vi "Vision Processing.vi"(4 "error in (no error)":errorcluster, 7 "Image Size":T5=enum."320x240") -> ()   [LabVIEW 2015]
uses:
  <vilib>/Rock Robotics/WPI/Camera/WPI_CameraImageSize.ctl
  <vilib>/Rock Robotics/WPI/Camera/WPI_CameraWhite Balance Values.ctl
  <vilib>/Rock Robotics/WPI/Camera/WPI_CameraExposure Values.ctl
  <vilib>/Rock Robotics/WPI/Camera/WPI_CameraFrameRate.ctl
  Vision Support Code/Camera Types.ctl
  Robot Global Data.vi
  <vilib>/vision/NI_Vision_Development_Module.lvlib
panel:
  out "Normalized Rect":T1
  out "Center":cluster{dbl, dbl}
  out "element":T2
  out "Highest Avg Score":dbl
  in  "Min Score Threshold":i32=75
  out "Detected Targets":T3(array[cluster]) {"Normalized Rect"."Numeric 5" format="%#_2g"; "Normalized Rect"."Numeric 3" format="%#_2g"; "Normalized Rect"."Numeric 2" format="%#_2g"; "Normalized Rect"."Numeric" format="%#_2g"}
  out "Sorted Particle Scores":T4(array[cluster]) {"Moment Factor" format="%#_3g"; "Aspect Ratio" format="%#_3g"; "Area to CH" format="%#_3g"; "X" format="%#_3g"; "Y" format="%#_3g"}
  in  "Display Original":bool=TRUE
  in  "Display Mask":bool=TRUE
  out "fps":dbl
  in  "Emphasize Limit Tests":bool=TRUE
  in  "Aspect Fudge Factor":dbl=1.0
  in  "Score Threshold":dbl=75.0
  out "ms to process":u32
  out "Qualified Particles":i32
  in  "LED Color":T6={"Hue"={111.0, 149.0}, "Sat"={35.0, 255.0}, "Val"={93.0, 255.0}} {"Hue" scale=0.0..255.0 scale format="%#_3g"}
  out "Masked":T7(plugin-control)
  out "Original Image":T7(plugin-control)
  # "NOTE:\nFor best results, lower the camera\nexposure."
  # "This is only the initial camera size.\nOther camera setup is done\non the diagram. Notice it is set\nonce before the loop but can be\nupdated within the loop if needed."
  # "Instructions:\nUse LED Color to threshold and build particles. Adjust calibration if needed.\nDisplays are very useful for debugging, but will slow down execution, so you\nmay want to disable once working.\nAnnotations show the rectangle and the scores from top to bottom.\nChange camera setting on diagram."
  # "Density Profile"
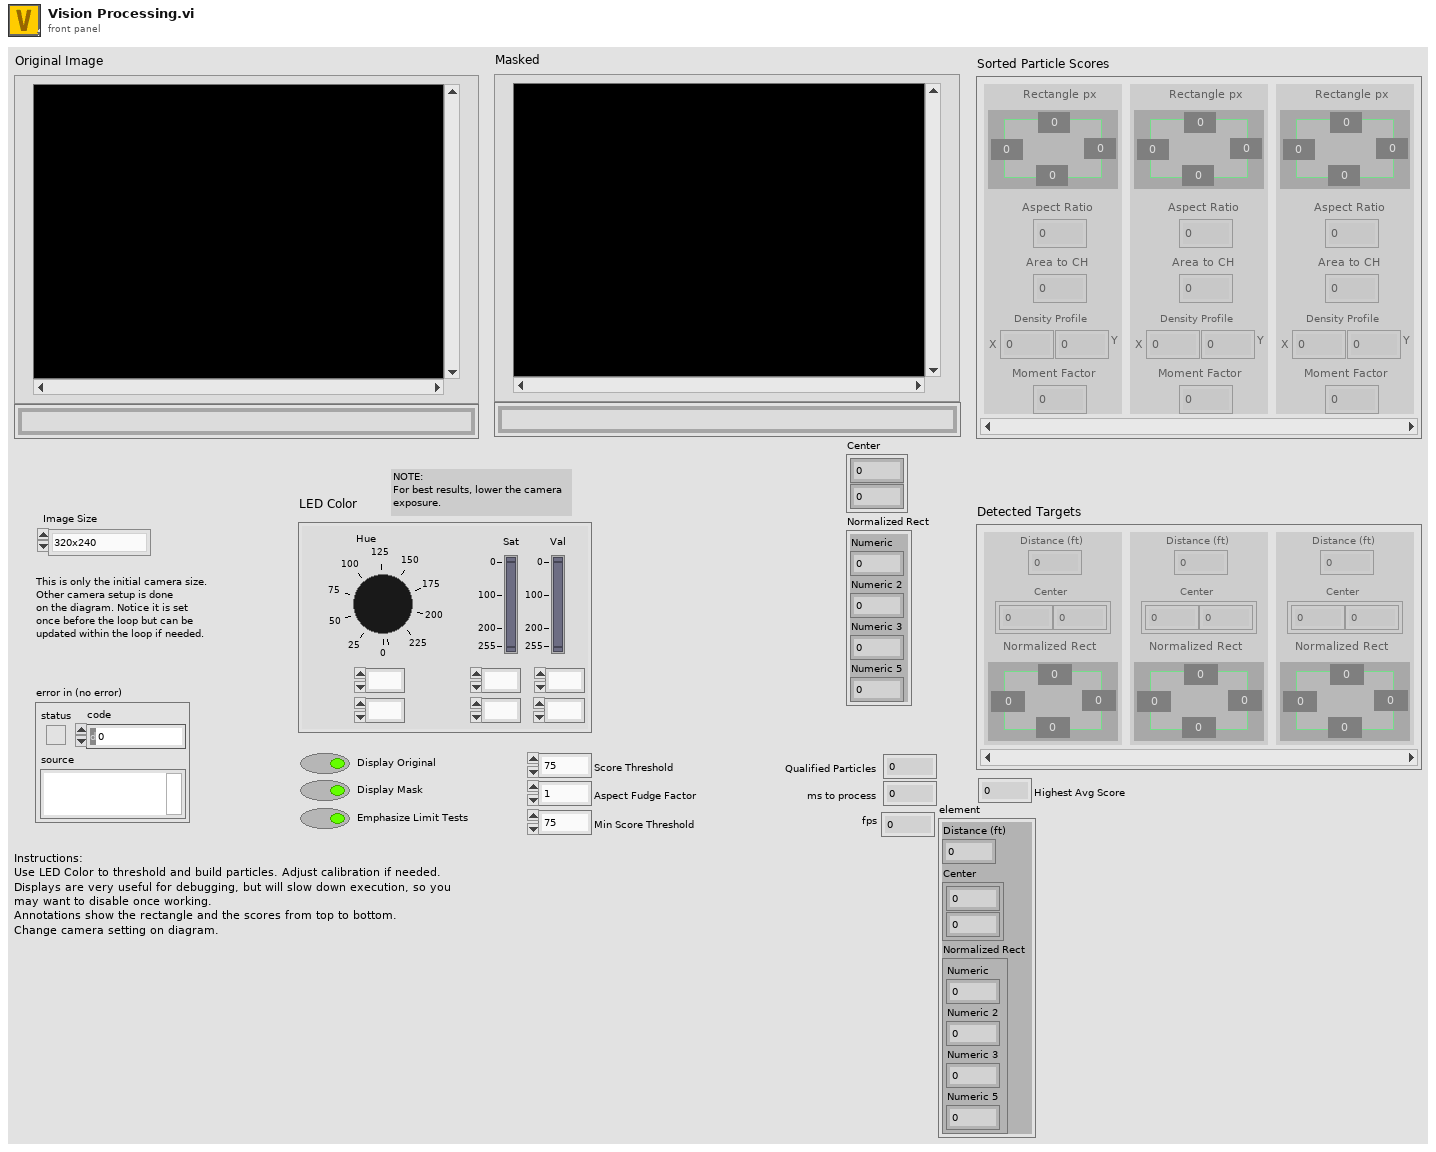
[diagram p1: front panel]
types:
  T1 = cluster{"Numeric":dbl, "Numeric 2":dbl, "Numeric 3":dbl, "Numeric 5":dbl}
  T2 = cluster{"Distance (ft)":dbl, "Center":cluster{dbl, dbl}, "Normalized Rect":cluster{"Numeric":dbl, "Numeric 2":dbl, "Numeric 3":dbl, "Numeric 5":dbl}}
  T3 = cluster{"Distance (ft)":dbl, "Center":cluster{dbl, dbl}, "Normalized Rect":cluster{"Numeric":dbl, "Numeric 2":dbl, "Numeric 3":dbl, "Numeric 5":dbl}}[]
  T4 = cluster{"Rectangle px":cluster{"Numeric":dbl, "Numeric 2":dbl, "Numeric 3":dbl, "Numeric 5":dbl}, "Aspect Ratio":dbl, "Area to CH":dbl, "X":dbl, "Y":dbl, "Moment Factor":dbl}[]
  T5 = typedef "WPI_CameraImageSize.ctl" = enum16{"640x480", "320x240", "160x120", "Custom"}
  T6 = cluster{"Hue":cluster{dbl, dbl}, "Sat":cluster{dbl, dbl}, "Val":cluster{dbl, dbl}}
  T7 = typedef "IMAQ Image.ctl" = refnum<image>
  T8 = typedef "WPI_CameraFrameRate.ctl" = u32
  T9 = typedef "WPI_CameraExposure Values.ctl" = enum16{"Auto", "Flicker-free 50 Hz", "Flicker-free 60 Hz", "Hold current", "Custom"}
  T10 = typedef "WPI_CameraWhite Balance Values.ctl" = enum16{"Auto", "Fixed indoor", "Fixed outdoor 1", "Fixed outdoor 2", "Fixed fluorescent 1", "Fixed fluorescent 2", "Hold current", "Custom"}
  T11 = typedef "Particle Parameters" = i32
  T12 = typedef "Image Type" = u32
  T13 = typedef "WPI_CameraDevRef.ctl" = cluster{"Camera Address":string, "CameraStatus":errorcluster}
  T14 = typedef "Camera Types.ctl" = enum16{"206", "1011", "1013", "MS HD3000 square", "MS HD3000 640x480"}
  T15 = cluster{"Bounding box":cluster{"left":dbl, "top":dbl, "right":dbl, "bottom":dbl}, "Aspect Ratio":dbl, "Area to CH":dbl, "X Mask":dbl, "Y Mask":dbl, "Moment":dbl}[]
  T16 = cluster{"Rectangle":cluster{"Numeric":dbl, "Numeric 2":dbl, "Numeric 3":dbl, "Numeric 5":dbl}, "L":dbl, "Area to CH":dbl, "X":dbl, "Y":dbl, "Moment Factor":dbl}[]
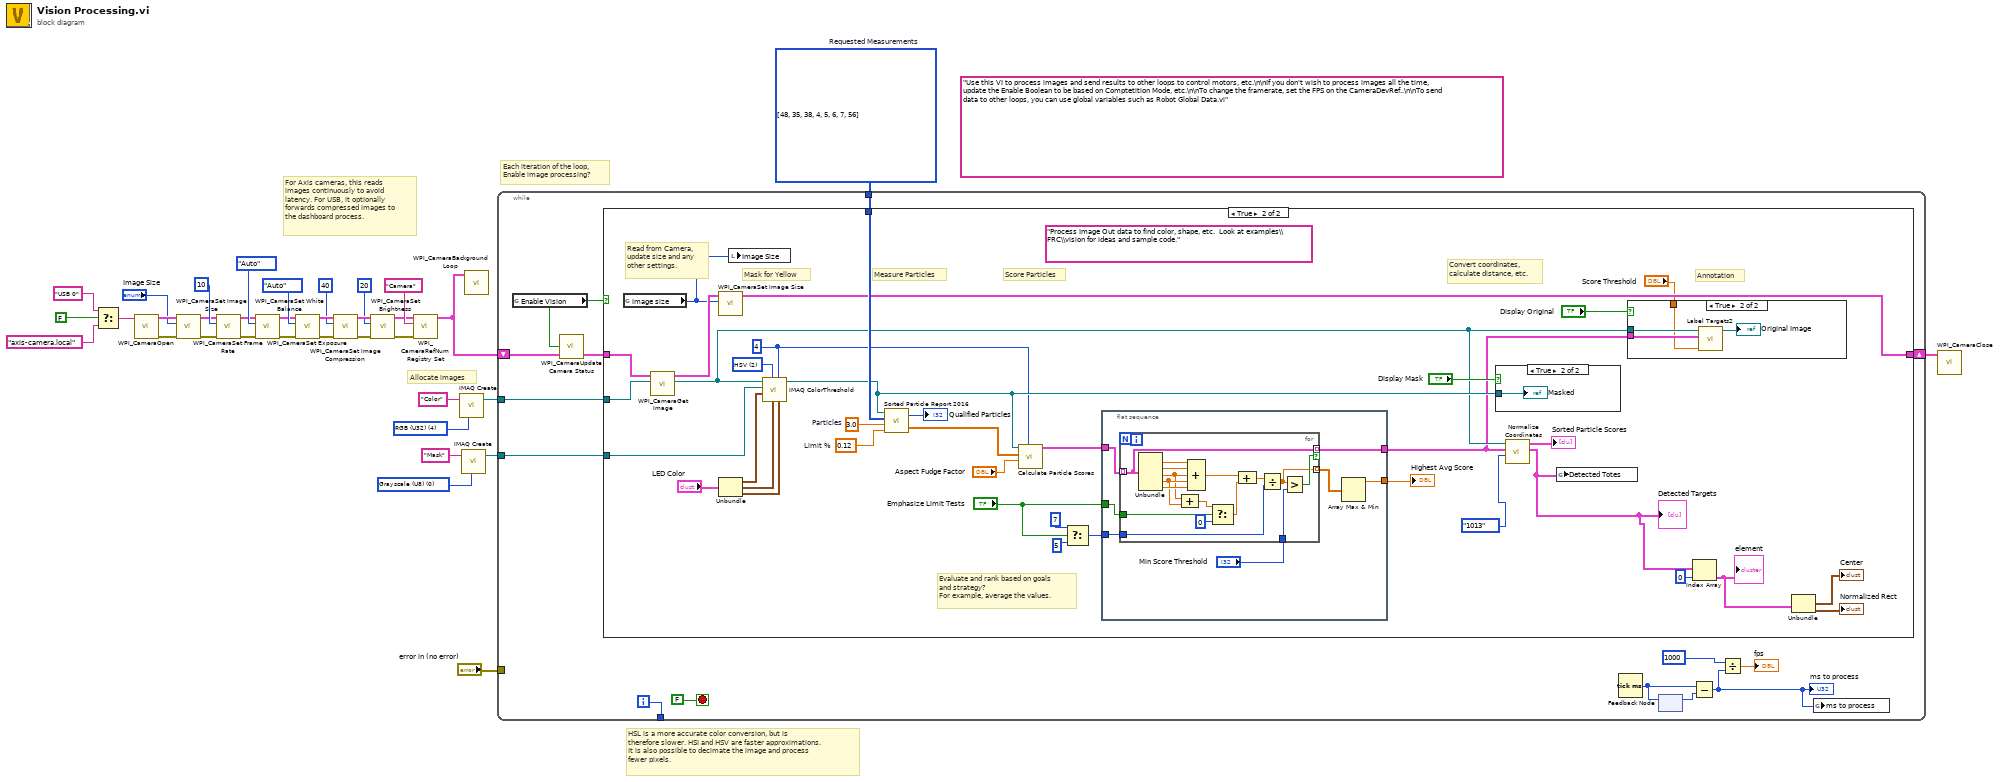
[diagram p0: block diagram]
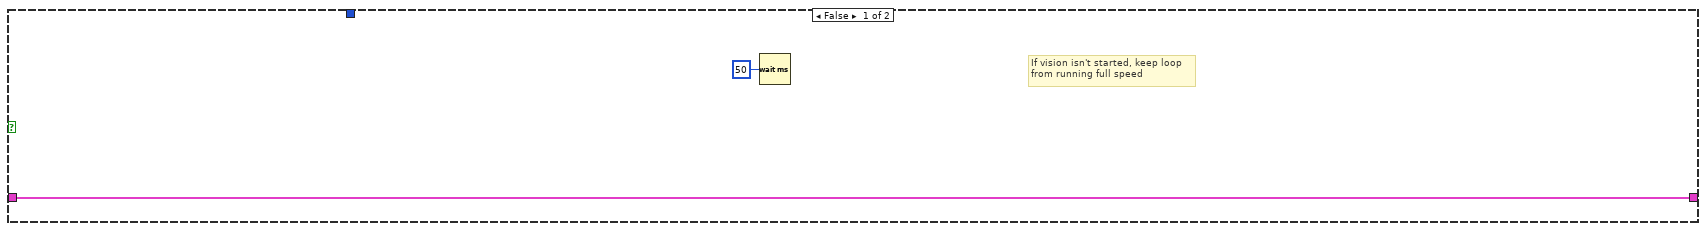
[diagram p2: hidden frame]
diagram:
  (unwired) "Use this VI to process images and send results to other loops to control motors, etc.\n\nIf you don't wish to process images all the time, update the Enable Boolean to be based on Comptetition Mode, etc.\n\nTo change the framerate, set the FPS on the CameraDevRef..\n\nTo send data to other loops, you can use global variables such as Robot Global Data.vi"
  w29 = T11[] [48, 35, 38, 4, 5, 6, 7, 56] items=["Center of Mass X", "Center of Mass Y", "First Pixel X", "First Pixel Y", "Bounding Rect Left", "Bounding Rect Top", "Bounding Rect Right", "Bounding Rect Bottom", "Max Feret Diameter Start X", "Max Feret Diameter Start Y", "Max Feret Diameter End X", "Max Feret Diameter End Y", "Max Horiz. Segment Length Left", "Max Horiz. Segment Length Right", "Max Horiz. Segment Length Row", "-", "Bounding Rect Width", "Bounding Rect Height", "Bounding Rect Diagonal", "Perimeter", "Convex Hull Perimeter", "Holes' Perimeter", "Max Feret Diameter", "Equivalent Ellipse Major Axis", "Equivalent Ellipse Minor Axis", "Equivalent Ellipse Minor Axis (Feret)", "Equivalent Rect Long Side", "Equivalent Rect Short Side", "Equivalent Rect Diagonal", "Equivalent Rect Short Side (Feret)", "Average Horiz. Segment Length", "Average Vert. Segment Length", "Hydraulic Radius", "Waddel Disk Diameter", "-", "Area", "Holes' Area", "Particle & Holes' Area", "Convex Hull Area", "Image Area", "-", "Number of Holes", "Number of Horiz. Segments", "Number of Vert. Segments", "-", "Orientation", "Max Feret Diameter Orientation", "-", "% Area/Image Area", "% Area/(Particle & Holes' Area)", "Ratio of Equivalent Ellipse Axes", "Ratio of Equivalent Rect Sides", "-", "Elongation Factor", "Compactness Factor", "Heywood Circularity Factor", "Type Factor", "-", "Sum X", "Sum Y", "Sum XX", "Sum XY", "Sum YY", "Sum XXX", "Sum XXY", "Sum XYY", "Sum YYY", "-", "Moment of Inertia XX", "Moment of Inertia XY", "Moment of Inertia YY", "Moment of Inertia XXX", "Moment of Inertia XXY", "Moment of Inertia XYY", "Moment of Inertia YYY", "Norm. Moment of Inertia XX", "Norm. Moment of Inertia XY", "Norm. Moment of Inertia YY", "Norm. Moment of Inertia XXX", "Norm. Moment of Inertia XXY", "Norm. Moment of Inertia XYY", "Norm. Moment of Inertia YYY", "Hu Moment 1", "Hu Moment 2", "Hu Moment 3", "Hu Moment 4", "Hu Moment 5", "Hu Moment 6", "Hu Moment 7"]  # Requested Measurements
  w32 = T12 0 items=["Grayscale (U8)", "Grayscale (I16)", "Grayscale (SGL)", "Complex (CSG)", "RGB (U32)", "HSL (U32)", "RGB (U64)", "Grayscale (U16)"] ("Image Type")
  w34 = T12 4 items=["Grayscale (U8)", "Grayscale (I16)", "Grayscale (SGL)", "Complex (CSG)", "RGB (U32)", "HSL (U32)", "RGB (U64)", "Grayscale (U16)"] ("Image Type")
  # "Each iteration of the loop,\nEnable image processing?"
  # "HSL is a more accurate color conversion, but is\ntherefore slower. HSI and HSV are faster approximations.\nIt is also possible to decimate the image and process\nfewer pixels."
  # "For Axis cameras, this reads\nimages continuously to avoid\nlatency. For USB, it optionally\nforwards compressed images to\nthe dashboard process."
  # "Allocate images"
  n1 = Select(t="USB 0" ("format string"), s=FALSE ("dot notation? (F)"), f="axis-camera.local" ("format string")) -> (s? t:f=w28:string)
  n2 = call <vilib>:"WPI_CameraOpen.vi"("Camera Address"=w28) -> ("error out"=w16:errorcluster, "CameraDevRef"=w15:T13)  [unwired: 1 in, 8 out]
  n3 = call <vilib>:"WPI_CameraSet Image Size.vi"("error in (no error)"=w16, "Image Size"="Image Size", "CameraDevRef"=w15) -> ("error out"=w17:errorcluster, "CameraDevRef Out"=w14:T13)  [unwired: 1 in, 6 out]
  n4 = call <vilib>:"WPI_CameraSet Frame Rate.vi"("error in (no error)"=w17, "Frame Rate (fps)"=T8 10, "CameraDevRef"=w14) -> ("error out"=w18:errorcluster, "CameraDevRef Out"=w12:T13)  [unwired: 7 out]
  n5 = call <vilib>:"WPI_CameraSet White Balance.vi"("error in (no error)"=w18, "White Balance"=WPI_CameraWhite_Balance_Values."Auto", "CameraDevRef"=w12) -> ("error out"=w19:errorcluster, "CameraDevRef Out"=w13:T13)  [unwired: 1 in, 6 out]
  n6 = call <vilib>:"WPI_CameraSet Exposure.vi"("error in (no error)"=w19, "Exposure"=WPI_CameraExposure_Values."Auto", "CameraDevRef"=w13) -> ("error out"=w20:errorcluster, "CameraDevRef Out"=w10:T13)  [unwired: 1 in, 6 out]
  n7 = call <vilib>:"WPI_CameraSet Image Compression.vi"("error in (no error)"=w20, "Compression"=40, "CameraDevRef"=w10) -> ("error out"=w21:errorcluster, "CameraDevRef Out"=w11:T13)  [unwired: 7 out]
  n8 = call <vilib>:"WPI_CameraSet Brightness.vi"("error in (no error)"=w21, "Brightness"=20, "CameraDevRef"=w11) -> ("error out"=w22:errorcluster, "CameraDevRef Out"=w1:T13)  [unwired: 7 out]
  n9 = call <vilib>:"WPI_CameraRefNum Registry Set.vi"("error in (no error)"=w22, "refnum name"="Camera", "CameraDevRef"=w1) -> ("CameraDevRef"=w6:T13)  [unwired: 1 in, 7 out]
  n10 = call "IMAQ Create"("Image Name"="Color", "Image Type"=w34) -> ("New Image"=w33:T7)  [unwired: 2 in, 2 out]
  n11 = call "IMAQ Create"("Image Name"="Mask", "Image Type"=w32) -> ("New Image"=w30:T7)  [unwired: 2 in, 2 out]
  n12 = call <vilib>:"WPI_CameraBackground Loop.vi"("CameraDevRef"=w6) -> ()  [unwired: 11 in]
  n13 = while {
    tunnel: w33 -> [w44]
    tunnel: w30 -> [w48]
    tunnel: w29 -> [w47]
    tunnel: "error in (no error)" -> [_]
    tunnel: [w43] -> _
    shift-right: [w39] -> w2
    shift-left: w6 -> [w41]
    i -> [w43]
    stop <- FALSE stop-if-true
    n14 = global read "Robot Global Data.vi" "Enable Vision"() -> (w42:bool)
    n15 = call <vilib>:"WPI_CameraUpdate Camera Status.vi"("CameraDevRef In"=w41, "Enable Vision"=w42) -> ("CameraDevRef Out"=w40:T13)  [unwired: 3 in]
    n16 = case shown="True" w42 {
      tunnel: w48 -> [_ w88]
      tunnel: w47 -> [_ w83]
      tunnel: w40 -> [w50 w79]
      tunnel: w44 -> [_ w78]
      tunnel: [w50 w76] -> w39
      frame False {
        # "If vision isn't started, keep loop\nfrom running full speed"
        n17 = Wait (ms)(milliseconds to wait=u32 50) -> ()  [unwired: 1 out]
      }
      frame True {
        w60 = 4 ("Replace Value")
        w73 = u16 2 items=["RGB", "HSL", "HSV", "HSI"] ("Color Mode")
        (unwired) "Process Image Out data to find color, shape, etc.  Look at examples\\FRC\\vision for ideas and sample code."
        w80 = 0.12  # Limit %
        w82 = 3.0  # Particles
        # "Evaluate and rank based on goals\nand strategy?\nFor example, average the values."
        # "Read from Camera,\nupdate size and any\nother settings."
        # "Measure Particles"
        # "Convert coordinates,\ncalculate distance, etc."
        # "Annotation"
        # "Score Particles"
        # "Mask for Yellow"
        n18 = global read "Robot Global Data.vi" "image size"() -> (w59:T5)
        n19 = call <vilib>:"WPI_CameraGet Image.vi"("Image"=w78, "CameraDevRef"=w79) -> ("Image Out"=w63:T7, "CameraDevRef Out"=w77:T13)  [unwired: 7 in, 1 out]
        n20 = call <vilib>:"WPI_CameraSet Image Size.vi"("Image Size"=w59, "CameraDevRef"=w77) -> ("CameraDevRef Out"=w76:T13)  [unwired: 2 in, 7 out]
        n21 = Unbundle("LED Color") -> ("Hue"=w87:cluster{dbl, dbl}, "Sat"=w86:cluster{dbl, dbl}, "Val"=w85:cluster{dbl, dbl})
        n22 = local write "Image Size"(w59) -> ()
        n23 = call "IMAQ ColorThreshold"("Blue or Luma or Val or Inten Range"=w85, "Replace Value"=w60, "Green or Sat Range"=w86, "Color Mode"=w73, "Red or Hue Range"=w87, "Image Dst"=w88, "Image Src"=w63) -> ("Image Dst Out"=w72:T7)  [unwired: 3 in, 1 out]
        n24 = call "Sorted Particle Report 2016.vi"("Min Area Size %"=w80, "Particle Count Limit"=w82, "Pixel Measurements"=w83, "Image in"=w72) -> ("Sorted Data"=w71:dbl[][], "Particles"=→"Qualified Particles":i32)
        n25 = call "Calculate Particle Scores.vi"("Pixel Value"=w60, "Aspect Fudge Factor"="Aspect Fudge Factor", "Sorted Data"=w71, "Image in"=w72) -> ("Scores"=w69:T15)  [unwired: 7 in]
        n26 = Select(t=7, s="Emphasize Limit Tests", f=5) -> (s? t:f=w66:i32)
        n27 = flat-sequence {
          tunnel: w69 -> [w99]
          tunnel: w66 -> [w97]
          tunnel: [w100] -> w65
          tunnel: [w94] -> w62
          tunnel: "Emphasize Limit Tests" -> [w98]
          frame #0 {
            n28 = for {
              tunnel: w99 -> [w114] mode=indexing
              tunnel: [w114] -> w94 mode=indexing if=w113
              tunnel: [w112] -> w95 mode=indexing
              tunnel: w97 -> [w111]
              tunnel: "Min Score Threshold" -> [w110]
              tunnel: w98 -> [w103]
              n29 = Unbundle(w114) -> ("Aspect Ratio"=w116:dbl, "Area to CH"=w115:dbl, "X Mask"=w105:dbl, "Y Mask"=w106:dbl, "Moment"=w107:dbl)  [unwired: 1 out]
              n30 = Compound Arithmetic op=ADD(w105, w106) -> (w104:dbl)
              n31 = Compound Arithmetic op=ADD(w116, w115, w105, w106, w107) -> (w109:dbl)
              n32 = Select(t=w104, s=w103, f=0) -> (s? t:f=w102:dbl)
              n33 = Compound Arithmetic op=ADD(w109, w102) -> (w108:dbl)
              n34 = Divide(x=w108, y=w111) -> (x/y=w112:dbl)
              n35 = Greater?(x=w112, y=w110) -> (0:w113:bool)
            }
            n36 = Array Max & Min(array=w95) -> (max value=w100:dbl)  [unwired: 3 out]
          }
        }
        n37 = case shown="True" "Display Mask" {
          tunnel: w72 -> [_ w93]
          frame False {
          }
          frame True {
            "Masked" <- w93
          }
        }
        n38 = call "Normalize Coordinates.vi"("Camera Type"=Camera_Types."1013", "Targets"=w62, "Image in"=w63) -> ("Found Targets"=w56:T3, "Sorted Scores"=→"Sorted Particle Scores":T16)  [unwired: 7 in]
        "Detected Targets" <- w56
        n39 = global write "Robot Global Data.vi" "Detected Totes"(w56) -> ()
        n40 = case shown="True" "Display Original" {
          tunnel: w63 -> [_ w92]
          tunnel: w62 -> [_ w90]
          tunnel: "Score Threshold" -> [_ w89]
          frame False {
          }
          frame True {
            n41 = call "Label Targets2.vi"("Score Threshold"=w89, "Targets"=w90, "Image in"=w92) -> ("Image out"=→"Original Image":T7)  [unwired: 8 in]
          }
        }
        n42 = Index Array(array=w56, index=0) -> (element=w54:T2)
        "element" <- w54
        n43 = Unbundle(w54) -> ("Center"=→"Center":cluster{dbl, dbl}, "Normalized Rect"=→"Normalized Rect":T1)  [unwired: 1 out]
        "Highest Avg Score" <- w65
      }
    }
    n44 = Tick Count (ms)() -> (millisecond timer value=w45:u32)
    n45 = feedback-in #1(w45) -> ()
    n46 = feedback #1() -> (w46:u32)  [unwired: 1 in]
    n47 = Subtract(x=w45, y=w46) -> (x-y=w38:u32)
    "ms to process" <- w38
    n48 = Divide(x=1000 ("Brightness"), y=w38) -> (x/y=→"fps":dbl)
    n49 = global write "Robot Global Data.vi" "ms to process"(w38) -> ()
  }
  n50 = call <vilib>:"WPI_CameraClose.vi"("CameraDevRef"=w2) -> ()  [unwired: 1 in, 10 out]
